vi "Water VFD Adjust.vi"(0 "PID Gains Cluster Ref":refnum<vi>, 1 "Accept Autotune":bool, 2 "Controller Toggle (Manual Mode)":bool, 3 "Valve Manual Adjust":dbl, 5 "Slide Refnum in":refnum<vi>, 7 "file (use dialog)":path, 9 "Desired Setpoint":dbl, 11 "PID gains":T2, 12 "Current Process Variable Value":dbl, 13 "autotune? (F)":bool, 14 "Reinitialize Controller":bool) -> (4 "output to valve":dbl, 6 "output to slide":dbl, 8 "tuning completed?":bool, 10 "plant parameters out":T1, 15 "PID gains out":T2)   [LabVIEW 2017]
uses:
  <vilib>/addons/control/pid/autopid.llb/PID autotuning parameters (FO).ctl
  <vilib>/addons/control/pid/NI_PID_autopid.lvlib
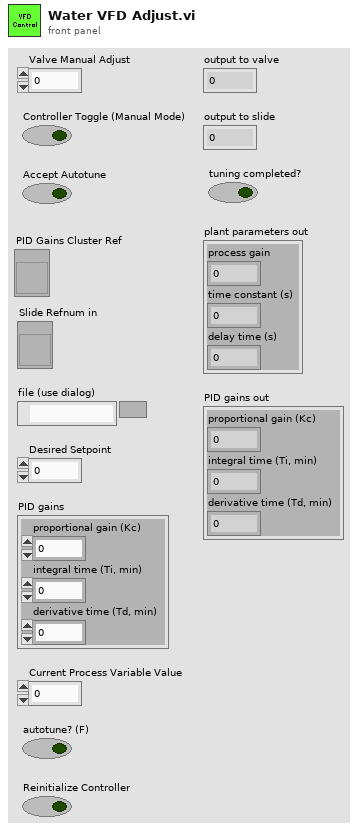
[diagram p1: front panel]
types:
  T1 = cluster{"process gain":dbl, "time constant (s)":dbl, "delay time (s)":dbl}
  T2 = cluster{"proportional gain (Kc)":dbl, "integral time (Ti, min)":dbl, "derivative time (Td, min)":dbl}
  T3 = typedef "NI_PID_autopid.lvlib/PID autotuning parameters (FO).ctl" = cluster{"type of controller":u16, "time constant factor":dbl, "step amplitude":dbl}
  T4 = enum8{"Enabled", "Disabled", "Disabled and Grayed Out"}
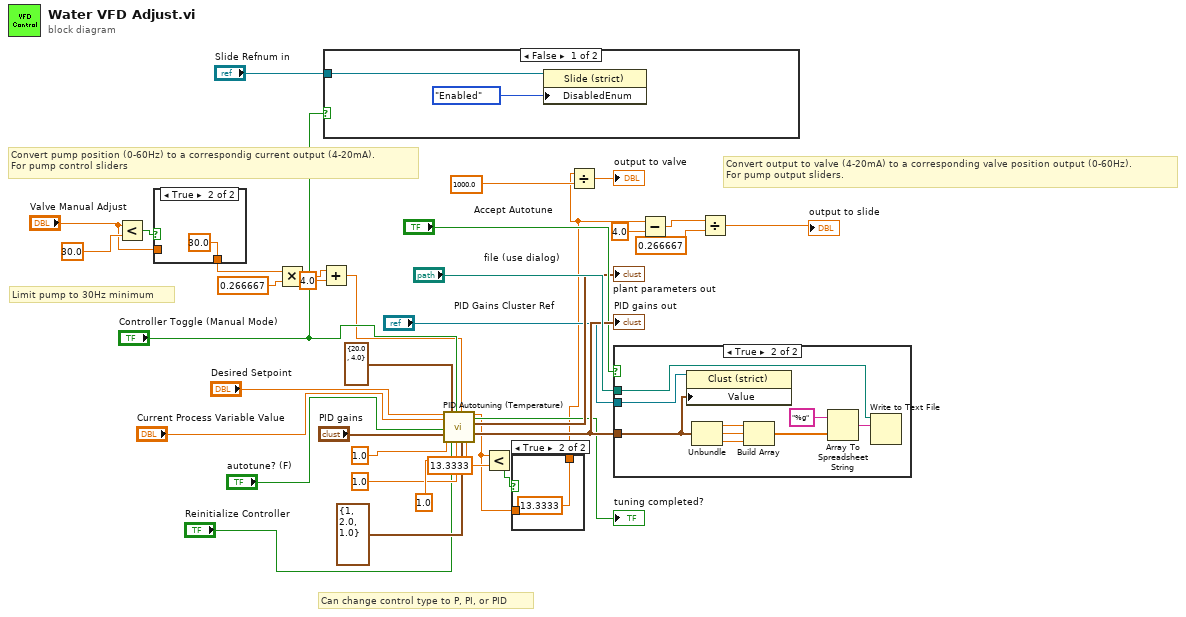
[diagram p0: block diagram]
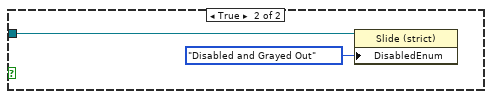
[diagram p5: hidden frame]
diagram:
  # "Limit pump to 30Hz minimum"
  # "Can change control type to P, PI, or PID"
  # "Convert output to valve (4-20mA) to a corresponding valve position output (0-60Hz). \nFor pump output sliders."
  # "Convert pump position (0-60Hz) to a correspondig current output (4-20mA). \nFor pump control sliders"
  n1 = Less?(x="Valve Manual Adjust", y=30.0) -> (x < y?=w7:bool)
  n2 = case shown="True" w7 {
    tunnel: [w37 30.0 ("y")] -> w6
    tunnel: "Valve Manual Adjust" -> [w37 _]
    frame False {
    }
    frame True {
    }
  }
  n3 = Multiply(x=w6, y=0.266667) -> (x*y=w17:dbl)
  n4 = Add(x=w17, y=4.0) -> (x+y=w15:dbl)
  n5 = case shown="False" "Controller Toggle (Manual Mode)" {
    tunnel: "Slide Refnum in" -> [w39 w42]
    frame False {
      n6 = property on="Property Node" class="Slide (strict)"(reference=w39, "DisabledEnum"=T4."Enabled" ("Disabled")) -> ()  [unwired: 1 in, 2 out]
    }
    frame True {
      n7 = property on="Property Node" class="Slide (strict)"(reference=w42, "DisabledEnum"=T4."Disabled and Grayed Out" ("Disabled")) -> ()  [unwired: 1 in, 2 out]
    }
  }
  n8 = call <vilib>:"PID Autotuning (Temperature).vi"("desired temperature"="Desired Setpoint", "measured temperature"="Current Process Variable Value", "autotune? (F)"="autotune? (F)", "PID gains in"="PID gains", "dt (s)"=1.0, "output range"=cluster{"output high":dbl, "output low":dbl} {"output high"=20.0, "output low"=4.0}, "reinitialize? (F)"="Reinitialize Controller", "auto? (T)"="Controller Toggle (Manual Mode)", "beta"=1.0, "manual control"=w15, "autotuning parameters"=T3 {"type of controller"=1, "time constant factor"=2.0, "step amplitude"=1.0}, "alpha"=1.0) -> ("output"=w1:dbl, "tuning completed?"=→"tuning completed?":bool, "plant parameters out"=→"plant parameters out":T1, "PID gains out"=w34:T2)  [unwired: 4 in]
  "PID gains out" <- w34
  n9 = Less?(x=w1, y=13.3333) -> (x < y?=w3:bool)
  n10 = case shown="True" w3 {
    tunnel: [w43 13.3333 ("y")] -> w2
    tunnel: w1 -> [w43 _]
    frame False {
    }
    frame True {
    }
  }
  n11 = Divide(x=w2, y=1000.0) -> (x/y=→"output to valve":dbl)
  n12 = case shown="True" "Accept Autotune" {
    tunnel: w34 -> [_ w53]
    tunnel: "file (use dialog)" -> [_ w46]
    tunnel: "PID Gains Cluster Ref" -> [_ w45]
    frame False {
    }
    frame True {
      n13 = property class="Clust (strict)"(reference=w45, "Value"=w53) -> ()  [unwired: 1 in, 2 out]
      n14 = Unbundle(w53) -> ("proportional gain (Kc)"=w52:dbl, "integral time (Ti, min)"=w51:dbl, "derivative time (Td, min)"=w50:dbl)
      n15 = Build Array(w52, w51, w50) -> (w49:dbl[])
      n16 = Array To Spreadsheet String(array=w49, 3:"%g" ("format string")) -> (spreadsheet string=w48:string)  [unwired: 1 in]
      n17 = Write to Text File(file (use dialog)=w46, text=w48) -> ()  [unwired: 2 in, 3 out]
    }
  }
  n18 = Subtract(x=w2, y=4.0) -> (x-y=w14:dbl)
  n19 = Divide(x=w14, y=0.266667) -> (x/y=→"output to slide":dbl)
